vi "openEvent.vi"(8 "error in (no error)":errorcluster, 11 "PixelflySettings in":refnum<class "PixelflySettings.lvclass">) -> (0 "error out":errorcluster, 3 "PixelflySettings out":refnum<class "PixelflySettings.lvclass">)   [LabVIEW 2011, in "Tools.lvlib" / "Settings.lvlib" / "PixelflySettings.lvclass"]
uses:
  PixelflySettings.lvclass
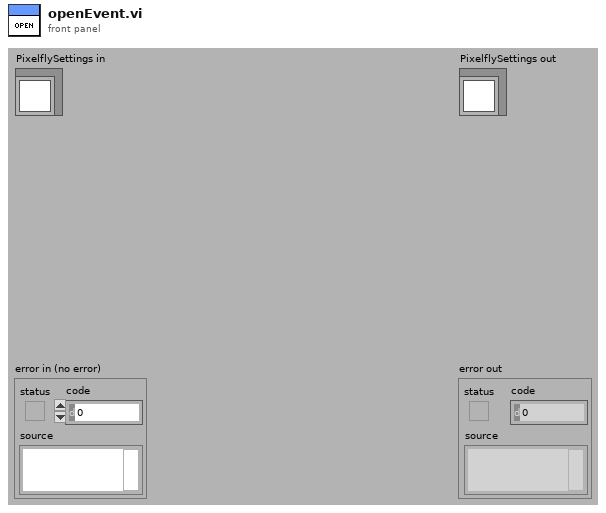
[diagram p1: front panel]
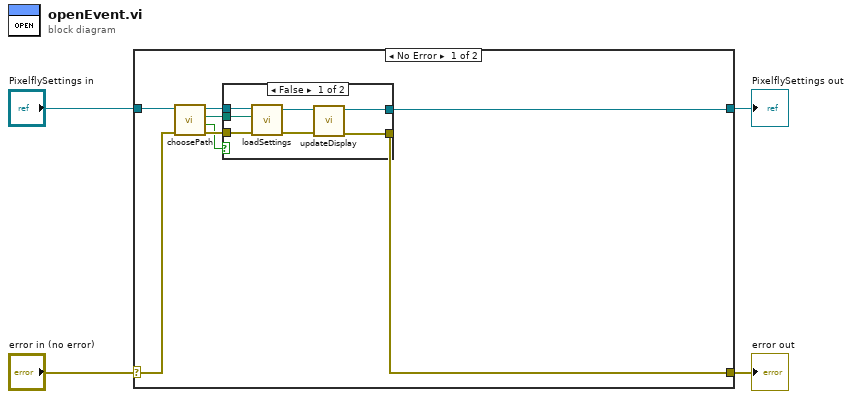
[diagram p0: block diagram]
diagram:
  n1 = case shown="No Error" "error in (no error)" {
    selector: "error in (no error)" -> [w9 w23]
    tunnel: [w6 w23] -> w3
    tunnel: [w7 w22] -> w1
    tunnel: "PixelflySettings in" -> [w10 w22]
    frame No Error {
      n2 = call "choosePath.vi"("error in (no error)"=w9, "PixelflySettings in"=w10) -> ("error out"=w8:errorcluster, "cancelled?"=w5:bool, "Path"=w11:path, "PixelflySettings out"=w12:refnum<class "PixelflySettings.lvclass">)  [unwired: 6 in]
      n3 = case shown="False" w5 {
        tunnel: w12 -> [w19 w21]
        tunnel: w11 -> [w18 _]
        tunnel: w8 -> [w17 w20]
        tunnel: [w14 w21] -> w7
        tunnel: [w13 w20] -> w6
        frame False {
          n4 = call-dynamic "loadSettings.vi"("error in (no error)"=w17, "Path"=w18, "PixelflySettings in"=w19) -> ("error out"=w15:errorcluster, "PixelflySettings out"=w16:refnum<class "PixelflySettings.lvclass">)  [unwired: 7 in]
          n5 = call "updateDisplay.vi"("error in (no error)"=w15, "PixelflySettings in"=w16) -> ("error out"=w13:errorcluster, "PixelflySettings out"=w14:refnum<class "PixelflySettings.lvclass">)  [unwired: 8 in]
        }
        frame True {
        }
      }
    }
    frame Error {
    }
  }
  "error out" <- w3
  "PixelflySettings out" <- w1
